vi "SetCh1Waveform.vi"(0 "object in":refnum<class "AD2_MSO_SDK.lvclass">, 1 "Ch1 waveform":waveform(dbl), 5 "error in (no error)":errorcluster) -> (14 "object out":refnum<class "AD2_MSO_SDK.lvclass">, 19 "error out":errorcluster)   [LabVIEW 2019, in "AD2_MSO_SDK.lvclass"]
uses:
  AD2_MSO_SDK.lvclass
  AD2_MSO_SDK.lvclass/AD2_MSO_SDK.ctl
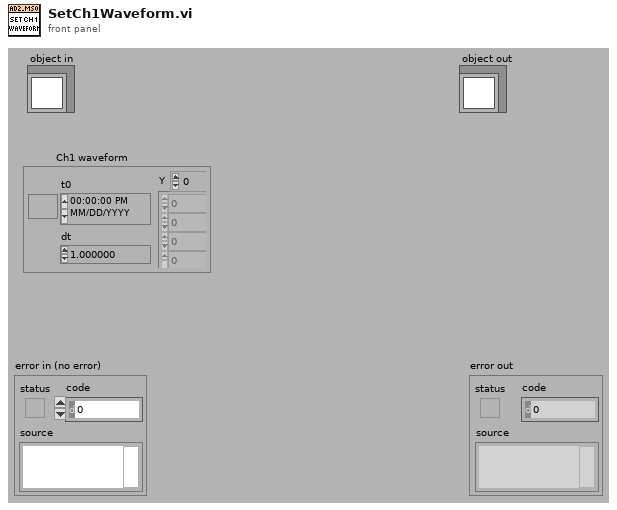
[diagram p1: front panel]
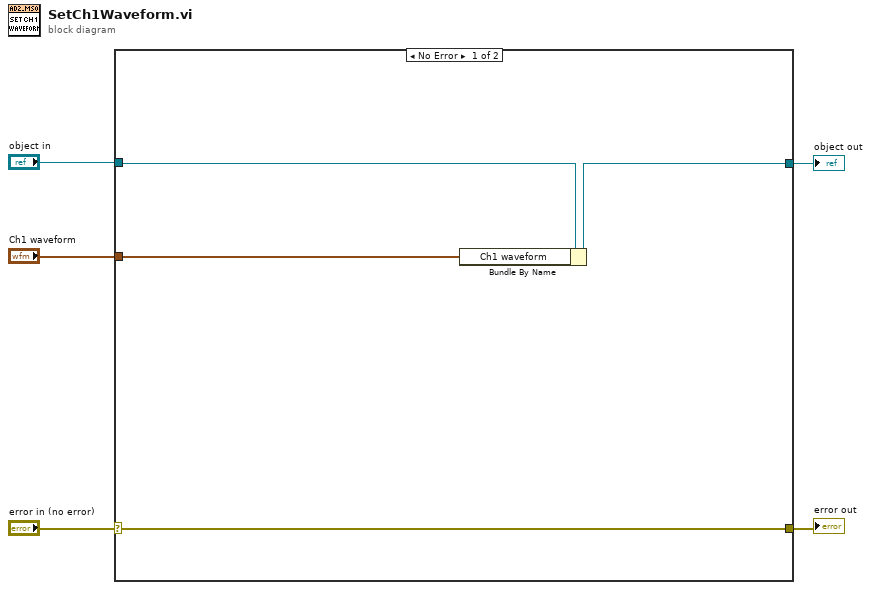
[diagram p0: block diagram]
diagram:
  n1 = case shown="No Error" "error in (no error)" {
    selector: "error in (no error)" -> [w8 w11]
    tunnel: [w8 w11] -> w4
    tunnel: [w6 w10] -> w2
    tunnel: "object in" -> [w7 w10]
    tunnel: "Ch1 waveform" -> [w9 _]
    frame No Error {
      n2 = Bundle By Name(cluster=w7, "Ch1 waveform"=w9) -> (w6:refnum<class "AD2_MSO_SDK.lvclass">)
    }
    frame Error {
    }
  }
  "error out" <- w4
  "object out" <- w2
